vi "error_bars.vi"(8 "y_error-":dbl[](array[numeric]), 9 "y_error+":dbl[](array[numeric]), 10 "y":dbl[](array[numeric]), 11 "x":dbl[](array[numeric])) -> (2 "error_bars":cluster{"dark_times_us":dbl[], dbl[]})   [LabVIEW 2018]
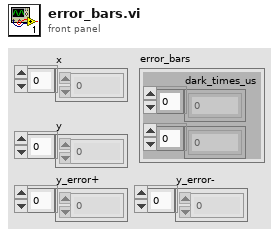
[diagram p1: front panel]
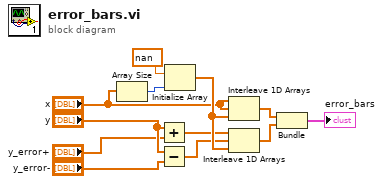
[diagram p0: block diagram]
diagram:
  n1 = Array Size(array="x") -> (size(s)=w5:i32)
  n2 = Add(x="y", y="y_error+") -> (x+y=w6:dbl[])
  n3 = Subtract(x="y", y="y_error-") -> (x-y=w7:dbl[])
  n4 = Initialize Array(nan ("element"), w5) -> (w10:dbl[])
  n5 = Interleave 1D Arrays("x", "x", w10) -> (w11:dbl[])
  n6 = Interleave 1D Arrays(w6, w7, w10) -> (w9:dbl[])
  n7 = Bundle(w11, w9) -> (→"error_bars":cluster{dbl[], dbl[]})  [unwired: 1 in]
